vi "Get Init Waiter.vi"(8 "Error In":errorcluster, 11 "Panel In":refnum<class "Panel.lvclass">) -> (0 "Error Out":errorcluster, 2 "Init Waiter":refnum<class "Init Waiter.lvclass">, 3 "Panel Out":refnum<class "Panel.lvclass">)   [LabVIEW 2023, in "Panel Actor.lvlib" / "Panel.lvlib" / "Panel.lvclass"]
doc: "Returns the Init Waiter for the panel.\n\n<B>Panel In:</B> Panel object in\n<B>Error In:</B> Describes error conditions that occur before this node runs.\n\n<B>Panel In:</B> Panel object out\n<B>Init Waiter:</B> Returns the Init Waiter object for the panel\n<B>Error Out:</B> Contains error information.\n----\nPlease see the following web address for additional documentation and tutorial information:\nhttp://www.mooregoodideas.com/mgi-panel-manager/\n\nAuthor: Derek Trepanier\n\nCopyright (c) 2018, Moore Good Ideas, Inc.\n\nAll rights reserved.\n\nRedistribution and use in source and binary forms, with or without modification, are permitted provided that the following conditions are met:\n\n * Redistributions of source code must retain the above copyright notice, this list of conditions and the following disclaimer.\n * Redistributions in binary form must reproduce the above copyright notice, this list of conditions and the following disclaimer in the documentation and/or other materials provided with the distribution.\n * Neither the name of Moore Good Ideas, Inc. nor the names of its contributors may be used to endorse or promote products derived from this software without specific prior written permission.\n\nTHIS SOFTWARE IS PROVIDED BY THE COPYRIGHT HOLDERS AND CONTRIBUTORS \"AS IS\" AND ANY EXPRESS OR IMPLIED WARRANTIES, INCLUDING, BUT NOT LIMITED TO, THE IMPLIED WARRANTIES OF MERCHANTABILITY AND FITNESS FOR A PARTICULAR PURPOSE ARE DISCLAIMED. IN NO EVENT SHALL THE COPYRIGHT OWNER OR CONTRIBUTORS BE LIABLE FOR ANY DIRECT, INDIRECT, INCIDENTAL, SPECIAL, EXEMPLARY, OR CONSEQUENTIAL DAMAGES (INCLUDING, BUT NOT LIMITED TO, PROCUREMENT OF SUBSTITUTE GOODS OR SERVICES; LOSS OF USE, DATA, OR PROFITS; OR BUSINESS INTERRUPTION) HOWEVER CAUSED AND ON ANY THEORY OF LIABILITY, WHETHER IN CONTRACT, STRICT LIABILITY, OR TORT (INCLUDING NEGLIGENCE OR OTHERWISE) ARISING IN ANY WAY OUT OF THE USE OF THIS SOFTWARE, EVEN IF ADVISED OF THE POSSIBILITY OF SUCH DAMAGE."
uses:
  Panel.lvclass
  Init Waiter/Init Waiter.lvclass
  Panel.lvclass/Panel.ctl
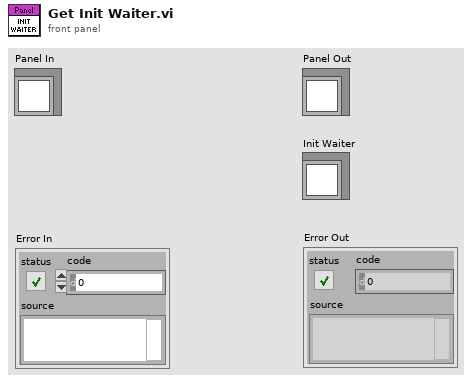
[diagram p1: front panel]
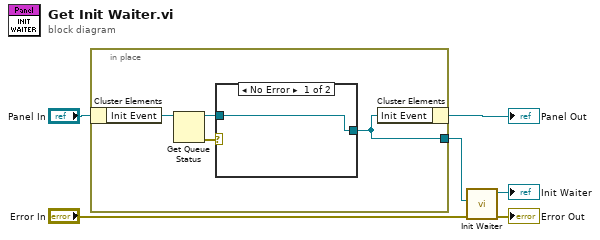
[diagram p0: block diagram]
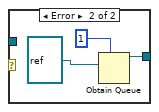
[diagram p2: hidden frame]
diagram:
  n1 = in-place {
    in-place-border: [w7] -> w4
    n2 = in-place-cluster #1("Panel In") -> ("Init Event"=w10:refnum<queue>)
    n3 = Get Queue Status(queue=w10) -> (queue out=w9:refnum<queue>, error out=w8:errorcluster)  [unwired: 2 in, 6 out]
    n4 = case shown="No Error" w8 {
      tunnel: [w11 w13] -> w7
      tunnel: w9 -> [w11 _]
      frame No Error {
      }
      frame Error {
        n5 = Obtain Queue(max queue size (-1, unlimited)=1, element data type=refnum<vi> refnum ("notification")) -> (queue out=w13:refnum<queue>)  [unwired: 3 in, 2 out]
      }
    }
    n6 = in-place-cluster #1("Init Event"=w7) -> (→"Panel Out":refnum<class "Panel.lvclass">)
  }
  n7 = call "Init Waiter.vi"("error in (no error)"="Error In", "Init Event"=w4) -> ("error out"=→"Error Out":errorcluster, "Init Waiter out"=→"Init Waiter":refnum<class "Init Waiter.lvclass">)  [unwired: 8 in]
